vi "Read Response.vi"(8 "error in (no error)":errorcluster, 11 "firebase in":refnum<class "firebase.lvclass">) -> (0 "error out":errorcluster, 2 "Succes Sign In":T1, 3 "firebase out":refnum<class "firebase.lvclass">)   [LabVIEW 2019, in "firebase.lvclass"]
uses:
  firebase.lvclass
  Success Sign In--cluster.ctl
  firebase.lvclass/firebase.ctl
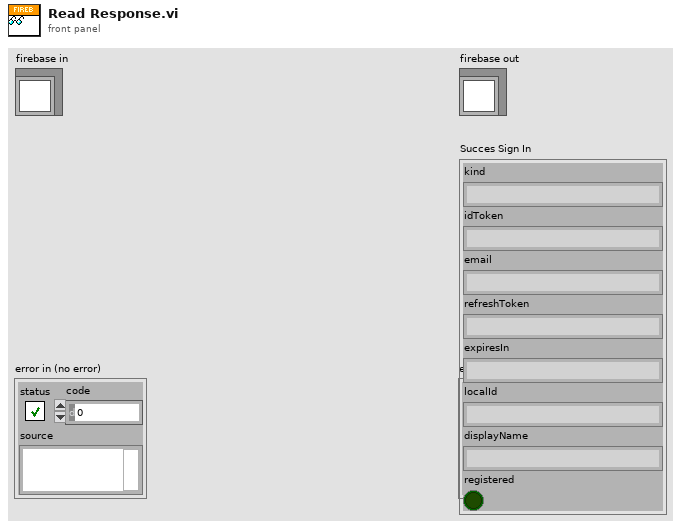
[diagram p1: front panel]
types:
  T1 = typedef "firebase.lvclass/Success Sign In--cluster.ctl" = cluster{"kind":string, "idToken":string, "email":string, "refreshToken":string, "expiresIn":string, "localId":string, "displayName":string, "registered":bool}
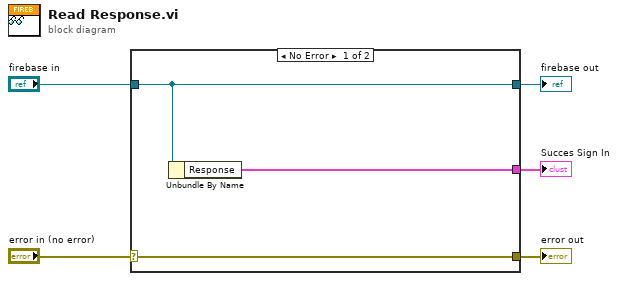
[diagram p0: block diagram]
diagram:
  n1 = case shown="No Error" "error in (no error)" {
    selector: "error in (no error)" -> [w8 w9]
    tunnel: [w8 w9] -> w4
    tunnel: [w7 w10] -> w2
    tunnel: "firebase in" -> [w7 w10]
    tunnel: [w6 _] -> w1
    frame No Error {
      n2 = Unbundle By Name(w7) -> ("Response"=w6:T1)
    }
    frame Error {
    }
  }
  "error out" <- w4
  "firebase out" <- w2
  "Succes Sign In" <- w1
